vi "Apply-median-filter.vi"(8 "error in":errorcluster, 9 "Corrected":T1[](array[typedef]), 11 "Median filter type":T2={"X Size"=3, "Y Size"=3, "Order #"=4}) -> (0 "error IO":errorcluster)   [LabVIEW 2013, in "CameraVision.lvlib" / "CV-Correction.lvclass"]
uses:
  CV-Correction.lvclass
  <vilib>/vision/Image Controls.llb/IMAQ Image.ctl
  <vilib>/vision/NI_Vision_Development_Module.lvlib
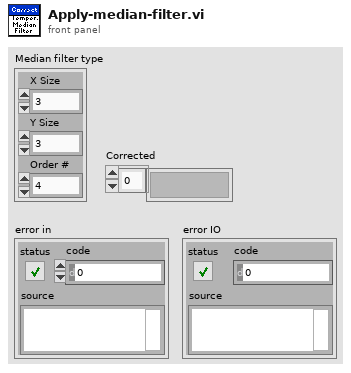
[diagram p1: front panel]
types:
  T1 = typedef "IMAQ Image.ctl" = refnum<image>
  T2 = cluster{"X Size":i32, "Y Size":i32, "Order #":i32}
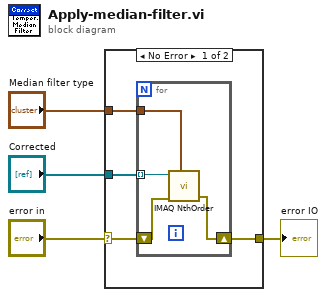
[diagram p0: block diagram]
diagram:
  n1 = case shown="No Error" "error in" {
    selector: "error in" -> [w8 w13]
    tunnel: "Corrected" -> [w7 _]
    tunnel: "Median filter type" -> [w6 _]
    tunnel: [w5 w13] -> w1
    frame No Error {
      n2 = for {
        tunnel: w7 -> [w10] mode=indexing
        tunnel: w6 -> [w9]
        shift-right: [w11] -> w5
        shift-left: w8 -> [w12]
        n3 = call "IMAQ NthOrder"("Image Src"=w10, "Size & Order #"=w9, "error in (no error)"=w12) -> ("error out"=w11:errorcluster)  [unwired: 4 in, 1 out]
      }
    }
    frame Error {
    }
  }
  "error IO" <- w1
